vi "Globals.vi"() -> ()   [LabVIEW 2014, in "GP22_TDC_Arduinoed.lvlib"]
uses:
  GP22_TDC_Arduinoed.lvlib
panel:
  out "Latest HF clock freq / Hz":dbl=4000000.0 format="%^#_6g"
  in  "Double res.":bool
  out "Latest LSB calibration / s":dbl format="%^#_4g"
  in  "Auto calibration":bool
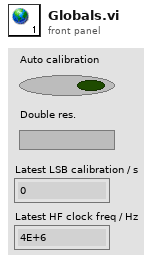
[diagram p1: front panel]
diagram:
